vi "UDT_loggingModule_Prerun.vi"() -> (3 "Unit Test Framework Results":T1)   [LabVIEW 2017]
doc: "Use this template to create a user-defined test VI. Define your test requirements and wire the results to the <b>Result (Test)</b> control. Do not modify the <b>Unit Test Framework Results</b> indicator."
uses:
  <vilib>/utf/common/utf_test_result_troll.ctl
  <vilib>/utf/common/utf_test_result.ctl
  <vilib>/utf/common/utf_test_result_failure.ctl
  <vilib>/utf/common/utf_test_comparison_operators.ctl
  <vilib>/utf/common/utf_vi_tag.ctl
  RT/loggingModule/Queue/TypeDefs/queueFGVState.ctl
  RT/loggingModule/Queue/TypeDefs/message.ctl
  <vilib>/Control Software Solutions Ltd/UTF Helper/SubVIs/UTF Variant Equals.vi
  RT/loggingModule/loggingModule.lvlib
  <vilib>/Control Software Solutions Ltd/UTF Helper/Unit Test Helper.lvlib
  <vilib>/utf/NI_UnitTestFramework.lvlib
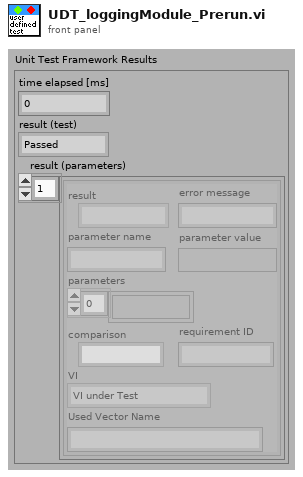
[diagram p1: front panel]
types:
  T1 = typedef "NI_UnitTestFramework.lvlib/utf_test_result_troll.ctl" = cluster{"time elapsed [ms]":u32, "result (test)":T2, "result (parameters)":T3[]}
  T2 = typedef "NI_UnitTestFramework.lvlib/utf_test_result.ctl" = enum16{"Passed", "Failed", "Error", "Skipped", "Not Processed"}
  T3 = typedef "NI_UnitTestFramework.lvlib/utf_test_result_failure.ctl" = cluster{"result":T2, "error message":string, "parameter name":string, "parameter value":variant, "parameters":variant[], "comparison":T4, "requirement ID":string, "VI":T5, "Used Vector Name":string}
  T4 = typedef "NI_UnitTestFramework.lvlib/utf_test_comparison_operators.ctl" = enum16{"=", "!=", ">", ">=", "<", "<=", "range", "symmetric tolerance", "asymmetric tolerance", "string contains", "string not contain", "array size", "string length", "array range", "by element", "array range (limit array)", "user-defined", "array contains", "array not contain", "vector length", "= (elm)", "!= (elm)", "= (case insensitive)", "!= (case insensitive)"}
  T5 = typedef "NI_UnitTestFramework.lvlib/utf_vi_tag.ctl" = enum16{"Setup VI", "VI under Test", "Teardown VI"}
  T6 = typedef "loggingModule.lvlib/queueFGVState.ctl" = enum16{"obtain", "enqueue low priority", "enqueue high priority", "dequeue", "release"}
  T7 = typedef "loggingModule.lvlib/message.ctl" = cluster{"calling module":string, "message":string, "data":variant}
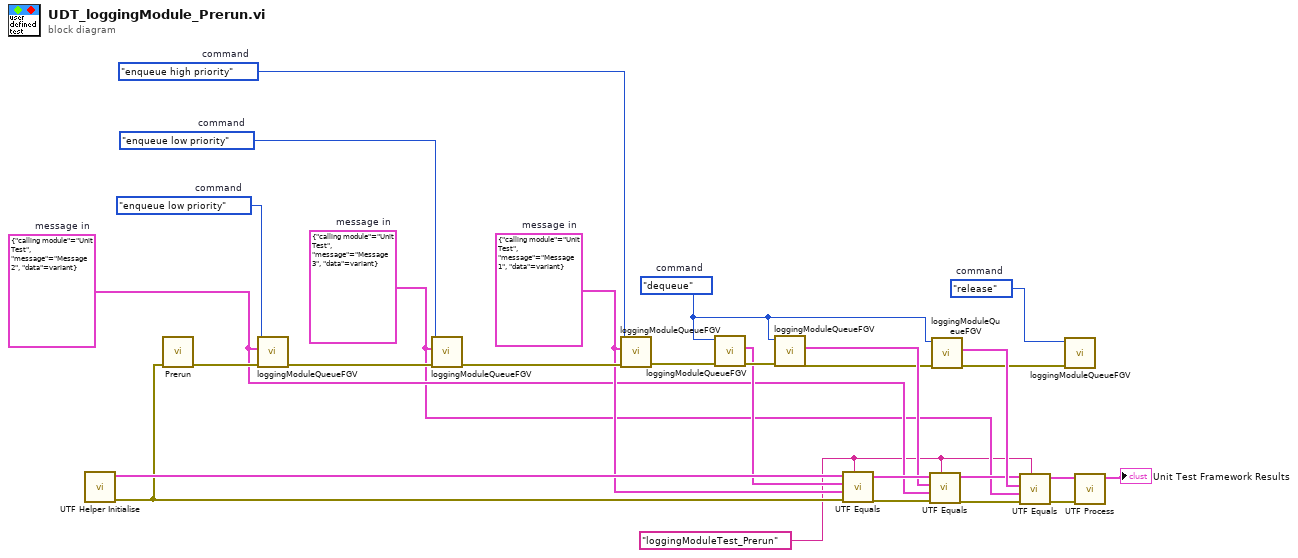
[diagram p0: block diagram]
diagram:
  w1 = "loggingModuleTest_Prerun"
  w2 = queueFGVState."release"  # command
  w10 = queueFGVState."dequeue"  # command
  w19 = T7 {"calling module"="Unit Test", "message"="Message 1", "data"=variant}  # message in
  w6 = T7 {"calling module"="Unit Test", "message"="Message 3", "data"=variant}  # message in
  w12 = T7 {"calling module"="Unit Test", "message"="Message 2", "data"=variant}  # message in
  w23 = queueFGVState."enqueue high priority"  # command
  w25 = queueFGVState."enqueue low priority"  # command
  w26 = queueFGVState."enqueue low priority"  # command
  n1 = call <vilib>:"UTF Helper Initialise.vi"() -> ("error out"=w20:errorcluster, "results array"=w21:T3[])  [unwired: 10 in]
  n2 = call "Prerun.vi"("error in (no error)"=w20) -> ("error out"=w27:errorcluster)  [unwired: 10 in]
  n3 = call "loggingModuleQueueFGV.vi"("error in (no error)"=w27, "message in"=w12, "command"=w26) -> ("error out"=w24:errorcluster)  [unwired: 7 in, 1 out]
  n4 = call "loggingModuleQueueFGV.vi"("error in (no error)"=w24, "message in"=w6, "command"=w25) -> ("error out"=w22:errorcluster)  [unwired: 7 in, 1 out]
  n5 = call "loggingModuleQueueFGV.vi"("error in (no error)"=w22, "message in"=w19, "command"=w23) -> ("error out"=w18:errorcluster)  [unwired: 7 in, 1 out]
  n6 = call "loggingModuleQueueFGV.vi"("error in (no error)"=w18, "command"=w10) -> ("error out"=w15:errorcluster, "message out"=w14:T7)  [unwired: 8 in]
  n7 = call "loggingModuleQueueFGV.vi"("error in (no error)"=w15, "command"=w10) -> ("error out"=w11:errorcluster, "message out"=w13:T7)  [unwired: 8 in]
  n8 = call-poly <vilib>:"UTF Equals.vi"("Parameter Name"=w1, "error in (no error)"=w20, "Test Value"=w19, "Input"=w14, "Input Results"=w21) -> ("error out"=w17:errorcluster, "Output Results"=w16:T3[])  [unwired: 5 in]
  n9 = call-poly <vilib>:"UTF Equals.vi"("Parameter Name"=w1, "error in (no error)"=w17, "Test Value"=w12, "Input"=w13, "Input Results"=w16) -> ("error out"=w7:errorcluster, "Output Results"=w8:T3[])  [unwired: 5 in]
  n10 = call "loggingModuleQueueFGV.vi"("error in (no error)"=w11, "command"=w10) -> ("error out"=w3:errorcluster, "message out"=w9:T7)  [unwired: 8 in]
  n11 = call-poly <vilib>:"UTF Equals.vi"("Parameter Name"=w1, "error in (no error)"=w7, "Test Value"=w6, "Input"=w9, "Input Results"=w8) -> ("error out"=w4:errorcluster, "Output Results"=w5:T3[])  [unwired: 5 in]
  n12 = call "loggingModuleQueueFGV.vi"("error in (no error)"=w3, "command"=w2) -> ()  [unwired: 8 in, 2 out]
  n13 = call <vilib>:"UTF Process.vi"("error in (no error)"=w4, "results array"=w5) -> ("Unit Test Framework Results"=→"Unit Test Framework Results":T1)  [unwired: 9 in]
